vi "SimulateCurrents.vi"(10 "Number of 6482s":i32=4, 11 "Number of 6485s":i32=1) -> (3 "Current Meter Data":T1)   [LabVIEW 2012]
uses:
  CurrentMeterData.ctl
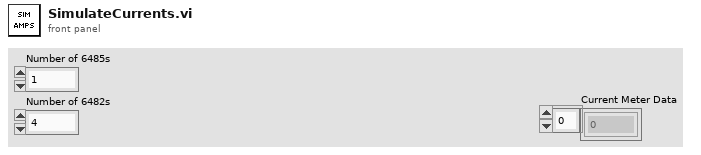
[diagram p1: front panel]
types:
  T1 = typedef "CurrentMeterData.ctl" = dbl[]
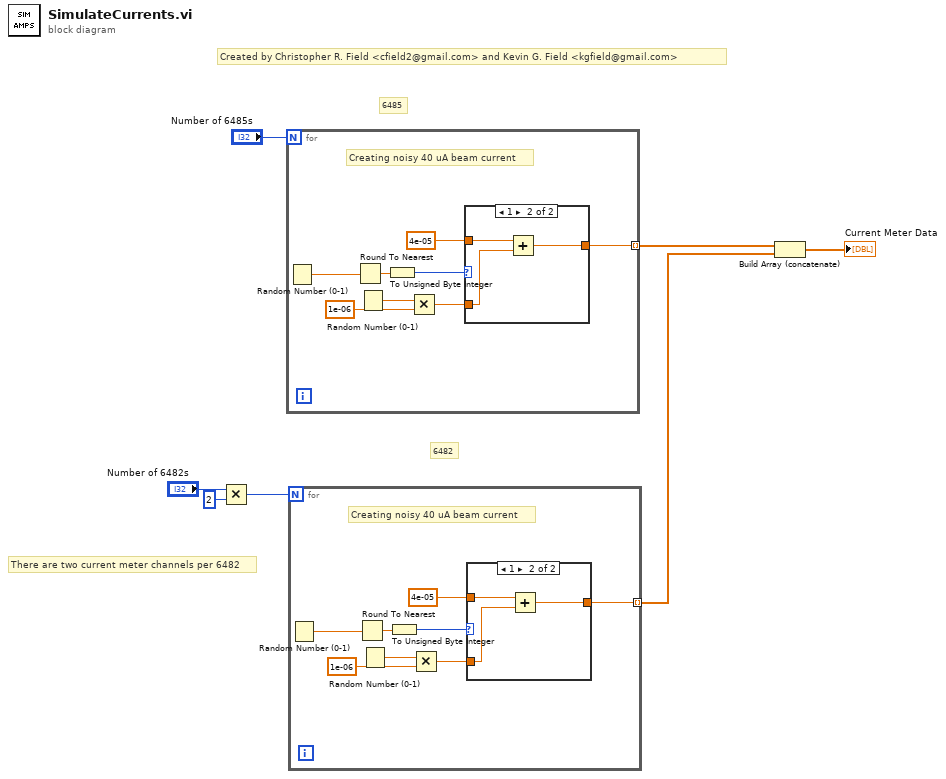
[diagram p0: block diagram]
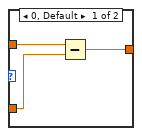
[diagram p2: hidden frame]
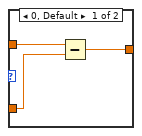
[diagram p3: hidden frame]
diagram:
  # "Created by Christopher R. Field <cfield2@gmail.com> and Kevin G. Field <kgfield@gmail.com>"
  # "There are two current meter channels per 6482"
  # "6482"
  # "6485"
  n1 = Multiply(x="Number of 6482s", y=2) -> (x*y=w2:i32)
  n2 = for {
    N: "Number of 6485s" -> [_]
    tunnel: [w8] -> w6 mode=indexing
    # "Creating noisy 40 uA beam current"
    n3 = Random Number (0-1)() -> (number: 0 to 1=w13:dbl)
    n4 = Round To Nearest(number=w13) -> (nearest integer value=w12:dbl)
    n5 = Random Number (0-1)() -> (number: 0 to 1=w15:dbl)
    n6 = To Unsigned Byte Integer(number=w12) -> (unsigned 8bit integer=w11:u8)
    n7 = Multiply(x=w15, y=1e-06) -> (x*y=w9:dbl)
    n8 = case shown="1" w11 {
      tunnel: 4e-05 -> [w18 w21]
      tunnel: w9 -> [w17 w20]
      tunnel: [w16 w19] -> w8
      frame 0, Default {
        n9 = Subtract(x=w18, y=w17) -> (x-y=w16:dbl)
      }
      frame 1 {
        n10 = Add(x=w21, y=w20) -> (x+y=w19:dbl)
      }
    }
  }
  n11 = for {
    N: w2 -> [_]
    tunnel: [w22] -> w5 mode=indexing
    # "Creating noisy 40 uA beam current"
    n12 = Random Number (0-1)() -> (number: 0 to 1=w27:dbl)
    n13 = Round To Nearest(number=w27) -> (nearest integer value=w26:dbl)
    n14 = Random Number (0-1)() -> (number: 0 to 1=w29:dbl)
    n15 = To Unsigned Byte Integer(number=w26) -> (unsigned 8bit integer=w25:u8)
    n16 = Multiply(x=w29, y=1e-06) -> (x*y=w23:dbl)
    n17 = case shown="1" w25 {
      tunnel: 4e-05 -> [w32 w35]
      tunnel: w23 -> [w31 w34]
      tunnel: [w30 w33] -> w22
      frame 0, Default {
        n18 = Subtract(x=w32, y=w31) -> (x-y=w30:dbl)
      }
      frame 1 {
        n19 = Add(x=w35, y=w34) -> (x+y=w33:dbl)
      }
    }
  }
  n20 = Build Array (concatenate)(w6, w5) -> (→"Current Meter Data":dbl[])
